vi "checkPauseTimeElapsed.vi"(8 "error in (no error)":errorcluster, 11 "Model in":refnum<class "Model.lvclass">) -> (0 "error out":errorcluster, 2 "pauseTimeHasElapsedIsTrue":bool, 3 "Model out":refnum<class "Model.lvclass">)   [LabVIEW 2013, in "Model.lvclass"]
uses:
  Model.lvclass
  Model.lvclass/Model.ctl
  ApplicationElements/TestMonitor/TestMonitor.lvclass
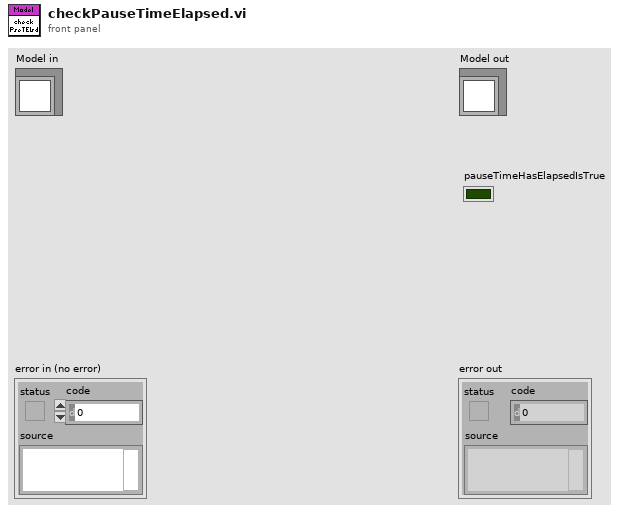
[diagram p1: front panel]
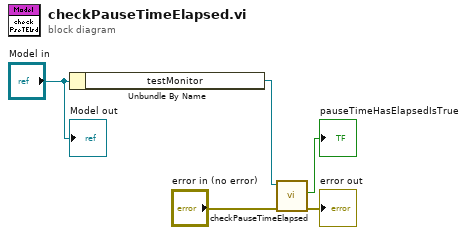
[diagram p0: block diagram]
diagram:
  n1 = Unbundle By Name("Model in") -> ("testMonitor"=w4:refnum<class "TestMonitor.lvclass">)
  n2 = call "checkPauseTimeElapsed.vi"("error in (no error)"="error in (no error)", "TestMonitor in"=w4) -> ("error out"=→"error out":errorcluster, "pauseTimeElapsedIsTrue"=→"pauseTimeHasElapsedIsTrue":bool)  [unwired: 7 in, 1 out]
  "Model out" <- "Model in"
